vi "myRIO_BRig_RT__Case_Exp_subState_LC__initTrial__v3.vi"(0 "input_dataCurrent":u16[](array[numeric]), 2 "input_dataLC":u16[](array[numeric]), 6 "input_spout":enum16{"Left", "Right"}(ring), 8 "input_dataTrial":u16[][](array[numeric])) -> (10 "output_dataTrial":u16[][](array[numeric]), 11 "output_LR_Wrong_Laser_l2":bool, 13 "output_LR_Reward_Laser_l2":bool, 14 "output_LR_Reward_Event_l1":bool, 15 "output_LR_Wrong_Event_l1":bool, 16 "output_LR_Reward_Laser_l1":bool, 17 "output_LR_Wrong_Laser_l1":bool, 18 "output_LR_Reward_Event_l2":bool, 19 "output_LR_Wrong_Event_l2":bool)   [LabVIEW 2014]
panel:
  in  "input_dataExp":u16[](array[numeric])
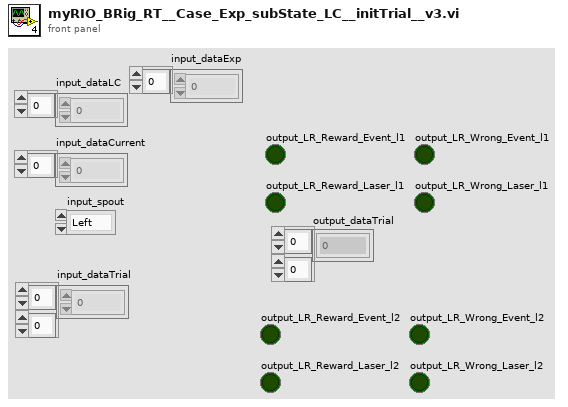
[diagram p1: front panel]
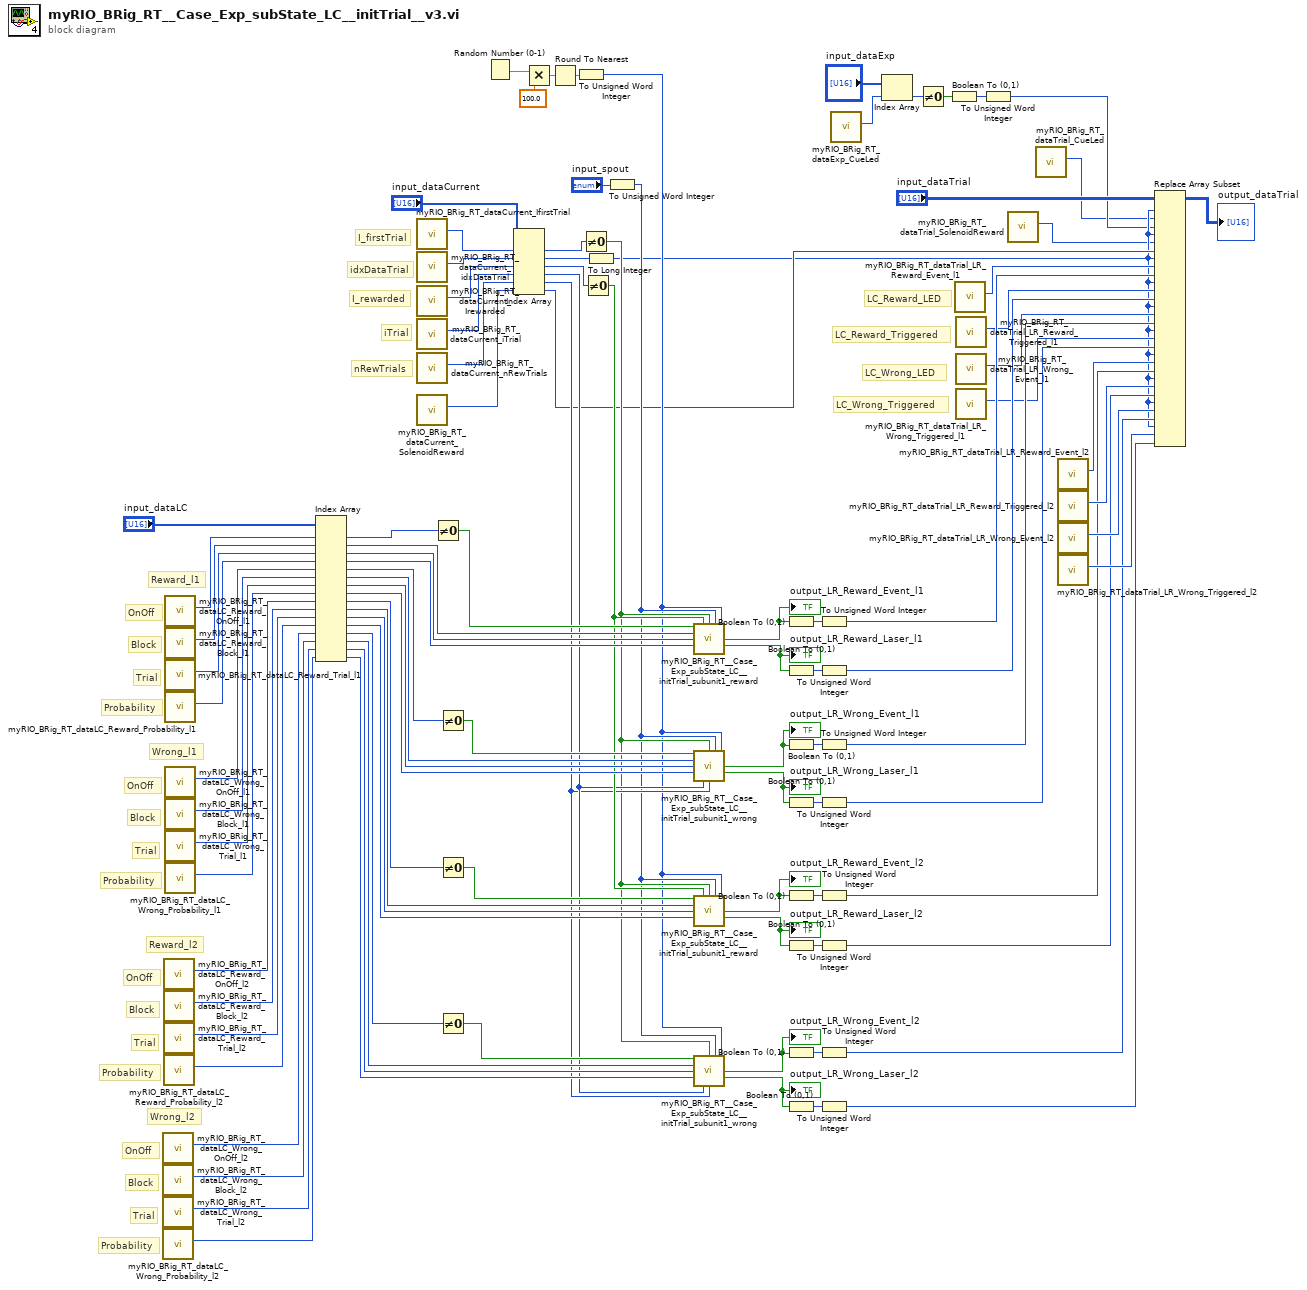
[diagram p0: block diagram]
diagram:
  # "Probability"
  # "Trial"
  # "Block"
  # "OnOff"
  # "Wrong_l2"
  # "Reward_l2"
  # "Probability"
  # "Trial"
  # "Block"
  # "OnOff"
  # "nRewTrials"
  # "iTrial"
  # "I_rewarded"
  # "LC_Wrong_Triggered"
  # "LC_Wrong_LED"
  # "LC_Reward_Triggered"
  # "LC_Reward_LED"
  # "idxDataTrial"
  # "Probability"
  # "Trial"
  # "Block"
  # "OnOff"
  # "Wrong_l1"
  # "I_firstTrial"
  # "Reward_l1"
  # "Probability"
  # "Trial"
  # "Block"
  # "OnOff"
  n1 = call "myRIO_BRig_RT_dataLC_Wrong_OnOff_l2.vi"() -> ("output_Wrong_OnOff_l2"=w58:i32)  [unwired: 11 in]
  n2 = call "myRIO_BRig_RT_dataLC_Wrong_Block_l2.vi"() -> ("output_Wrong_Block_l2"=w57:i32)  [unwired: 11 in]
  n3 = call "myRIO_BRig_RT_dataLC_Wrong_Trial_l2.vi"() -> ("output_Wrong_Trial_l2"=w56:i32)  [unwired: 11 in]
  n4 = call "myRIO_BRig_RT_dataLC_Wrong_Probability_l2.vi"() -> ("output_Wrong_Probability_l2"=w55:i32)  [unwired: 11 in]
  n5 = call "myRIO_BRig_RT_dataLC_Reward_OnOff_l2.vi"() -> ("output_Reward_OnOff_l2"=w62:i32)  [unwired: 11 in]
  n6 = call "myRIO_BRig_RT_dataLC_Reward_Block_l2.vi"() -> ("output_Reward_Block_l2"=w61:i32)  [unwired: 11 in]
  n7 = call "myRIO_BRig_RT_dataLC_Reward_Trial_l2.vi"() -> ("output_Reward_Trial_l2"=w60:i32)  [unwired: 11 in]
  n8 = call "myRIO_BRig_RT_dataLC_Reward_Probability_l2.vi"() -> ("output_Reward_Probability_l2"=w59:i32)  [unwired: 11 in]
  n9 = call "myRIO_BRig_RT_dataLC_Reward_OnOff_l1.vi"() -> ("output_Reward_OnOff_l1"=w101:i32)  [unwired: 11 in]
  n10 = call "myRIO_BRig_RT_dataLC_Reward_Block_l1.vi"() -> ("output_Reward_Block_l1"=w100:i32)  [unwired: 11 in]
  n11 = call "myRIO_BRig_RT_dataLC_Reward_Trial_l1.vi"() -> ("output_Reward_Trial_l1"=w99:i32)  [unwired: 11 in]
  n12 = call "myRIO_BRig_RT_dataLC_Reward_Probability_l1.vi"() -> ("output_Reward_Probability_l1"=w98:i32)  [unwired: 11 in]
  n13 = call "myRIO_BRig_RT_dataLC_Wrong_OnOff_l1.vi"() -> ("output_Wrong_OnOff_l1"=w90:i32)  [unwired: 11 in]
  n14 = call "myRIO_BRig_RT_dataLC_Wrong_Block_l1.vi"() -> ("output_Wrong_Block_l1"=w91:i32)  [unwired: 11 in]
  n15 = call "myRIO_BRig_RT_dataLC_Wrong_Trial_l1.vi"() -> ("output_Wrong_Trial_l1"=w92:i32)  [unwired: 11 in]
  n16 = call "myRIO_BRig_RT_dataLC_Wrong_Probability_l1.vi"() -> ("output_Wrong_Probability_l1"=w93:i32)  [unwired: 11 in]
  n17 = Index Array(array="input_dataLC", index #1=w101, index #2=w100, index #3=w99, index #4=w98, index #5=w90, index #6=w91, index #7=w92, index #8=w93, index #9=w62, index #10=w61, index #11=w60, index #12=w59, index #13=w58, index #14=w57, index #15=w56, index #16=w55) -> (element #1=w97:u16, element #2=w47:u16, element #3=w46:u16, element #4=w45:u16, element #5=w88:u16, element #6=w41:u16, element #7=w40:u16, element #8=w39:u16, element #9=w50:u16, element #10=w35:u16, element #11=w34:u16, element #12=w33:u16, element #13=w49:u16, element #14=w28:u16, element #15=w27:u16, element #16=w26:u16)
  n18 = call "myRIO_BRig_RT_dataCurrent_IfirstTrial.vi"() -> ("output_I_firstTrial"=w95:i32)  [unwired: 11 in]
  n19 = call "myRIO_BRig_RT_dataCurrent_idxDataTrial.vi"() -> ("output_idxDataTrial"=w87:i32)  [unwired: 11 in]
  n20 = call "myRIO_BRig_RT_dataCurrent_Irewarded.vi"() -> ("output_I_rewarded"=w71:i32)  [unwired: 11 in]
  n21 = call "myRIO_BRig_RT_dataCurrent_iTrial.vi"() -> ("output_iTrial"=w69:i32)  [unwired: 11 in]
  n22 = call "myRIO_BRig_RT_dataCurrent_nRewTrials.vi"() -> ("output_nRewTrials"=w68:i32)  [unwired: 11 in]
  n23 = call "myRIO_BRig_RT_dataCurrent_SolenoidReward.vi"() -> ("output_SolenoidReward"=w67:i32)  [unwired: 11 in]
  n24 = Not Equal To 0?(x=w97) -> (x != 0?=w48:bool)
  n25 = Not Equal To 0?(x=w88) -> (x != 0?=w42:bool)
  n26 = Not Equal To 0?(x=w50) -> (x != 0?=w36:bool)
  n27 = Not Equal To 0?(x=w49) -> (x != 0?=w29:bool)
  n28 = Random Number (0-1)() -> (number: 0 to 1=w63:dbl)
  n29 = Index Array(array="input_dataCurrent", index #1=w95, index #2=w87, index #3=w71, index #4=w69, index #5=w68, index #6=w67) -> (element #1=w94:u16, element #2=w86:u16, element #3=w70:u16, element #4=w25:u16, element #5=w24:u16, element #6=w18:u16)
  n30 = Multiply(x=w63, y=100.0) -> (x*y=w64:dbl)
  n31 = Round To Nearest(number=w64) -> (nearest integer value=w65:dbl)
  n32 = To Unsigned Word Integer(number=w65) -> (unsigned 16bit integer=w21:u16)
  n33 = Not Equal To 0?(x=w94) -> (x != 0?=w23:bool)
  n34 = Not Equal To 0?(x=w70) -> (x != 0?=w32:bool)
  n35 = To Long Integer(number=w86) -> (32bit integer=w9:i32)
  n36 = To Unsigned Word Integer(number="input_spout") -> (unsigned 16bit integer=w22:u16)
  n37 = call "myRIO_BRig_RT__Case_Exp_subState_LC__initTrial_subunit1_reward.vi"("input_LR_OnOff"=w48, "input_I_rewarded"=w32, "input_I_firstTrial"=w23, "input_spout"=w22, "input_randomNumber"=w21, "input_LR_Block"=w47, "input_LR_Trial"=w46, "input_LR_Probability"=w45) -> ("output_LR_Event"=w44:bool, "output_LR_Laser"=w43:bool)  [unwired: 6 in]
  "output_LR_Reward_Laser_l1" <- w43
  "output_LR_Reward_Event_l1" <- w44
  n38 = call "myRIO_BRig_RT__Case_Exp_subState_LC__initTrial_subunit1_wrong.vi"("input_LR_OnOff"=w42, "input_I_firstTrial"=w23, "input_spout"=w22, "input_randomNumber"=w21, "input_LR_Block"=w41, "input_LR_Trial"=w40, "input_LR_Probability"=w39, "input_iTrial"=w25, "input_nRewTrials"=w24) -> ("output_LR_Event"=w38:bool, "output_LR_Laser"=w37:bool)  [unwired: 5 in]
  "output_LR_Wrong_Laser_l1" <- w37
  "output_LR_Wrong_Event_l1" <- w38
  n39 = call "myRIO_BRig_RT__Case_Exp_subState_LC__initTrial_subunit1_reward.vi"("input_LR_OnOff"=w36, "input_I_rewarded"=w32, "input_I_firstTrial"=w23, "input_spout"=w22, "input_randomNumber"=w21, "input_LR_Block"=w35, "input_LR_Trial"=w34, "input_LR_Probability"=w33) -> ("output_LR_Event"=w31:bool, "output_LR_Laser"=w30:bool)  [unwired: 6 in]
  "output_LR_Reward_Laser_l2" <- w30
  "output_LR_Reward_Event_l2" <- w31
  n40 = call "myRIO_BRig_RT__Case_Exp_subState_LC__initTrial_subunit1_wrong.vi"("input_LR_OnOff"=w29, "input_I_firstTrial"=w23, "input_spout"=w22, "input_randomNumber"=w21, "input_LR_Block"=w28, "input_LR_Trial"=w27, "input_LR_Probability"=w26, "input_iTrial"=w25, "input_nRewTrials"=w24) -> ("output_LR_Event"=w20:bool, "output_LR_Laser"=w19:bool)  [unwired: 5 in]
  "output_LR_Wrong_Laser_l2" <- w19
  "output_LR_Wrong_Event_l2" <- w20
  n41 = Boolean To (0,1)(Boolean=w44) -> (0, 1=w82:i16)
  n42 = Boolean To (0,1)(Boolean=w43) -> (0, 1=w80:i16)
  n43 = Boolean To (0,1)(Boolean=w38) -> (0, 1=w76:i16)
  n44 = Boolean To (0,1)(Boolean=w37) -> (0, 1=w73:i16)
  n45 = Boolean To (0,1)(Boolean=w31) -> (0, 1=w54:i16)
  n46 = Boolean To (0,1)(Boolean=w30) -> (0, 1=w53:i16)
  n47 = Boolean To (0,1)(Boolean=w20) -> (0, 1=w52:i16)
  n48 = Boolean To (0,1)(Boolean=w19) -> (0, 1=w51:i16)
  n49 = To Unsigned Word Integer(number=w82) -> (unsigned 16bit integer=w81:u16)
  n50 = To Unsigned Word Integer(number=w80) -> (unsigned 16bit integer=w78:u16)
  n51 = To Unsigned Word Integer(number=w76) -> (unsigned 16bit integer=w75:u16)
  n52 = To Unsigned Word Integer(number=w73) -> (unsigned 16bit integer=w72:u16)
  n53 = To Unsigned Word Integer(number=w54) -> (unsigned 16bit integer=w13:u16)
  n54 = To Unsigned Word Integer(number=w53) -> (unsigned 16bit integer=w12:u16)
  n55 = To Unsigned Word Integer(number=w52) -> (unsigned 16bit integer=w11:u16)
  n56 = To Unsigned Word Integer(number=w51) -> (unsigned 16bit integer=w10:u16)
  n57 = call "myRIO_BRig_RT_dataExp_CueLed.vi"() -> ("output_CueLed"=w7:i32)  [unwired: 11 in]
  n58 = Index Array(array="input_dataExp", index=w7) -> (element=w6:u16)
  n59 = Not Equal To 0?(x=w6) -> (x != 0?=w5:bool)
  n60 = Boolean To (0,1)(Boolean=w5) -> (0, 1=w4:i16)
  n61 = call "myRIO_BRig_RT_dataTrial_LR_Reward_Event_l1.vi"() -> ("output_LR_Reward_Event_l1"=w83:i32)  [unwired: 11 in]
  n62 = call "myRIO_BRig_RT_dataTrial_LR_Reward_Triggered_l1.vi"() -> ("output_LR_Reward_Triggered_l1"=w79:i32)  [unwired: 11 in]
  n63 = call "myRIO_BRig_RT_dataTrial_LR_Wrong_Event_l1.vi"() -> ("output_LR_Wrong_Event_l1"=w77:i32)  [unwired: 11 in]
  n64 = call "myRIO_BRig_RT_dataTrial_LR_Wrong_Triggered_l1.vi"() -> ("output_LR_Wrong_Triggered_l1"=w74:i32)  [unwired: 11 in]
  n65 = To Unsigned Word Integer(number=w4) -> (unsigned 16bit integer=w3:u16)
  n66 = call "myRIO_BRig_RT_dataTrial_SolenoidReward.vi"() -> ("output_SolenoidReward"=w1:i32)  [unwired: 11 in]
  n67 = call "myRIO_BRig_RT_dataTrial_CueLed.vi"() -> ("output_CueLed"=w2:i32)  [unwired: 11 in]
  n68 = call "myRIO_BRig_RT_dataTrial_LR_Reward_Event_l2.vi"() -> ("output_LR_Reward_Event_l2"=w17:i32)  [unwired: 11 in]
  n69 = call "myRIO_BRig_RT_dataTrial_LR_Reward_Triggered_l2.vi"() -> ("output_LR_Reward_Triggered_l2"=w16:i32)  [unwired: 11 in]
  n70 = call "myRIO_BRig_RT_dataTrial_LR_Wrong_Event_l2.vi"() -> ("output_LR_Wrong_Event_l2"=w15:i32)  [unwired: 11 in]
  n71 = call "myRIO_BRig_RT_dataTrial_LR_Wrong_Triggered_l2.vi"() -> ("output_LR_Wrong_Triggered_l2"=w14:i32)  [unwired: 11 in]
  n72 = Replace Array Subset(array="input_dataTrial", new element #1=w3, index (row) #1=w9, index (col) #1=w2, new element #2=w18, index (row) #2=w9, index (col) #2=w1, new element #3=w81, index (row) #3=w9, index (col) #3=w83, new element #4=w78, index (row) #4=w9, index (col) #4=w79, new element #5=w75, index (row) #5=w9, index (col) #5=w77, new element #6=w72, index (row) #6=w9, index (col) #6=w74, new element #7=w13, index (row) #7=w9, index (col) #7=w17, new element #8=w12, index (row) #8=w9, index (col) #8=w16, new element #9=w11, index (row) #9=w9, index (col) #9=w15, new element #10=w10, index (row) #10=w9, index (col) #10=w14) -> (→"output_dataTrial":u16[][])
